vi "PhotonPNPResult_unpack.vi"(9 "StartByte":i32, 11 "RawData":u8[](array[numeric])) -> (1 "NextByte":i32, 3 "PNP_Result":T1={"IsPresent"=FALSE, "bestReprojErr"=0.0, "altReprojErr"=0.0, "ambiguity"=0.0, "Best"={"TRANSLATION3D"={"X"=0.0, "Y"=0.0, "Z"=0.0}, "ROTATION3D"={"Q_quaternion"={"R"=1.0, "V"=[0.0, 0.0, 0.0]}}, "XF"=FALSE}, "Alt"={"TRANSLATION3D"={"X"=0.0, "Y"=0.0, "Z"=0.0}, "ROTATION3D"={"Q_quaternion"={"R"=1.0, "V"=[0.0, 0.0, 0.0]}}, "XF"=FALSE}} {"Alt"."TRANSLATION3D"."Z" format="%14.3f"; "Alt"."TRANSLATION3D"."Y" format="%14.3f"; "Alt"."TRANSLATION3D"."X" format="%14.3f"; "Best"."TRANSLATION3D"."Z" format="%14.3f"; "Best"."TRANSLATION3D"."Y" format="%14.3f"; "Best"."TRANSLATION3D"."X" format="%14.3f"})   [LabVIEW 2019, in "PhotonVisionLib.lvlib"]
doc: "Internal function to parse the data for each PNP_Result returned by PhotonCamera_GetLatestResult.\n\nInputs:\n - RawData -- Byte array containing the data to parse.\n - StartingByte -- Index into raw data to start parsing. First byte is index 0.\n\nOutputs:\n - PNP_Result -- Parsed PNP_Result cluster."
uses:
  PhotonVisionLib.lvlib
  TypeDef/PhotonPNPResultType.ctl
  <vilib>/Rock Robotics/WPI/ThirdParty/JAS_Junk/TrajLib/TypeDef/TRANSFORM3D.ctl
  <vilib>/Rock Robotics/WPI/ThirdParty/JAS_Junk/TrajLib/TypeDef/TRANSLATION3D.ctl
  <vilib>/Rock Robotics/WPI/ThirdParty/JAS_Junk/TrajLib/TypeDef/ROTATION3D.ctl
  <vilib>/Rock Robotics/WPI/ThirdParty/JAS_Junk/TrajLib/TypeDef/QUATERNION.ctl
  <vilib>/Rock Robotics/WPI/ThirdParty/JAS_Junk/TrajLib/VI/Transform3d_Create_Trans3dRot3d.vi
  <vilib>/Rock Robotics/WPI/ThirdParty/JAS_Junk/TrajLib/VI/Translation3d_Create.vi
  <vilib>/Rock Robotics/WPI/ThirdParty/JAS_Junk/TrajLib/VI/Rotation3d_Create_Quaternion.vi
  <vilib>/Rock Robotics/WPI/ThirdParty/JAS_Junk/TrajLib/VI/Quaternion_New.vi
  <vilib>/Rock Robotics/WPI/ThirdParty/JAS_Junk/TrajLib/VI/Quaternion_Normalize.vi
  <vilib>/Rock Robotics/WPI/ThirdParty/JAS_Junk/TrajLib/VI/Quaternion_New_Default.vi
  <vilib>/Rock Robotics/WPI/ThirdParty/JAS_Junk/TrajLib/Trajectory_Library.lvlib
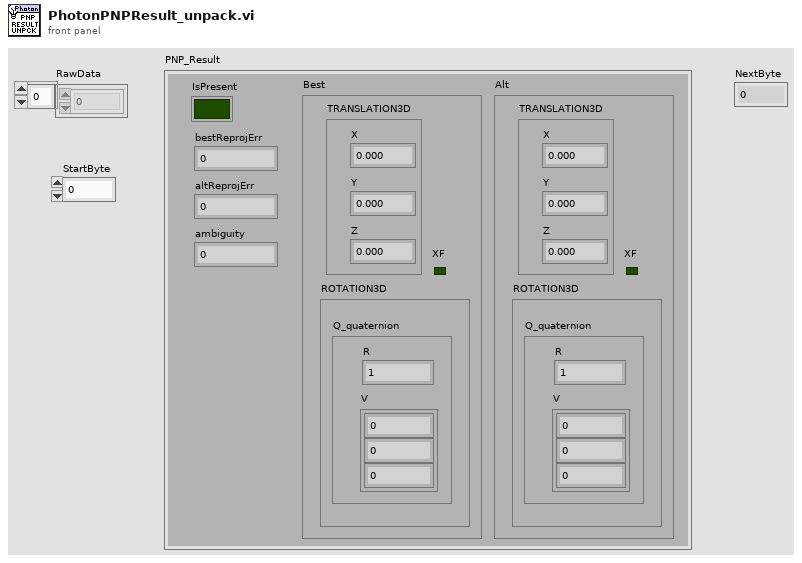
[diagram p1: front panel]
types:
  T1 = typedef "PhotonVisionLib.lvlib/PhotonPNPResultType.ctl" = cluster{"IsPresent":bool, "bestReprojErr":dbl, "altReprojErr":dbl, "ambiguity":dbl, "Best":T2, "Alt":T2}
  T2 = typedef "Trajectory_Library.lvlib/TRANSFORM3D.ctl" = cluster{"TRANSLATION3D":T3, "ROTATION3D":T4, "XF":bool}
  T3 = typedef "Trajectory_Library.lvlib/TRANSLATION3D.ctl" = cluster{"X":dbl, "Y":dbl, "Z":dbl}
  T4 = typedef "Trajectory_Library.lvlib/ROTATION3D.ctl" = cluster{"Q_quaternion":T5}
  T5 = typedef "Trajectory_Library.lvlib/QUATERNION.ctl" = cluster{"R":dbl, "V":dbl[]}
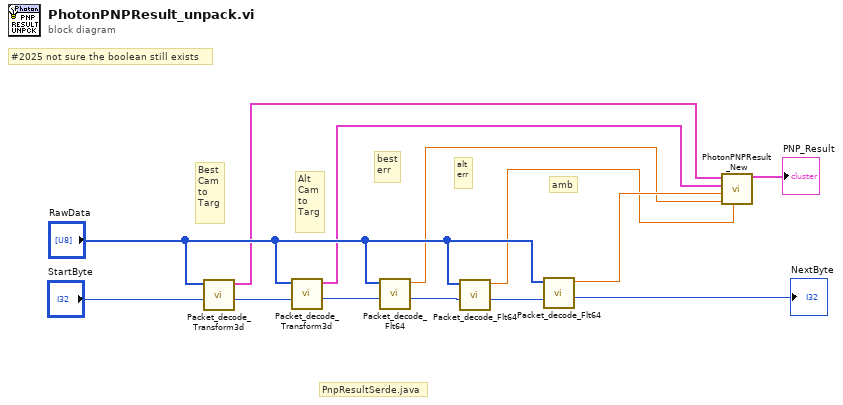
[diagram p0: block diagram]
diagram:
  # "PnpResultSerde.java"
  # "amb"
  # "alt\nerr"
  # "best\nerr"
  # "Alt\nCam\nto\nTarg"
  # "Best\nCam\nto\nTarg"
  # "#2025 not sure the boolean still exists"
  n1 = call "Packet_decode_Transform3d.vi"("NextByte in"="StartByte", "RawData"="RawData") -> ("NextByte out"=w8:i32, "Transform3d"=w7:T2)  [unwired: 6 in]
  n2 = call "Packet_decode_Transform3d.vi"("NextByte in"=w8, "RawData"="RawData") -> ("NextByte out"=w9:i32, "Transform3d"=w6:T2)  [unwired: 6 in]
  n3 = call "Packet_decode_Flt64.vi"("StartByte"=w9, "RawData"="RawData") -> ("NextByte"=w5:i32, "Flt64_Value"=w2:dbl)  [unwired: 8 in]
  n4 = call "Packet_decode_Flt64.vi"("StartByte"=w5, "RawData"="RawData") -> ("NextByte"=w4:i32, "Flt64_Value"=w1:dbl)  [unwired: 8 in]
  n5 = call "Packet_decode_Flt64.vi"("StartByte"=w4, "RawData"="RawData") -> ("NextByte"=→"NextByte":i32, "Flt64_Value"=w3:dbl)  [unwired: 8 in]
  n6 = call "PhotonPNPResult_New.vi"("altReprojErr"=w1, "bestReprojErr"=w2, "ambiguity"=w3, "Alt"=w6, "Best"=w7) -> ("PNP_Result"=→"PNP_Result":T1)  [unwired: 6 in]
